vi "PH_IEEE1394Camera.PC Write Attribute.vi"(0 "i ref out":refnum<vi>, 1 "Attribute Name":string="N/A", 2 "Wanted Num":dbl, 3 "Wanted String":string="N/A", 4 "Wanted Bool":bool, 5 "error out":errorcluster) -> (14 "i ref out":refnum<vi>, 19 "error out":errorcluster)   [LabVIEW 2014, in "PH_IEEE1394Camera.lvlib"]
doc: "By this VI the cam attribute of Ibnterest is written to the hardware if the cam is off."
uses:
  PH_IEEE1394Camera.lvlib
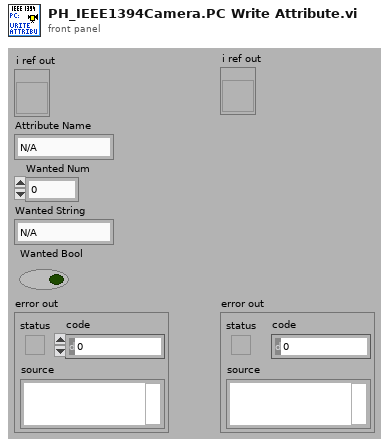
[diagram p1: front panel]
types:
  T1 = typedef "PH_IEEE1394Camera.lvlib/PH_IEEE1394Camera.i attribute.ctl" = cluster{"Gui Refs":cluster{"Brightness":refnum<vi>, "Shutter":refnum<vi>, "Gain":refnum<vi>, "Center of Gravity":refnum<vi>, "Supported Video Modes":refnum<vi>, "Trigger Polarity":refnum<vi>, "Trigger Mode":refnum<vi>, "Trigger Timeout":refnum<vi>, "Bit Depth":refnum<vi>, "Video Mode":refnum<vi>, "Top":refnum<vi>, "Bottom":refnum<vi>, "Left":refnum<vi>, "Right":refnum<vi>, "Set ROI to Maximum":refnum<vi>, "Camera Details":refnum<vi>, "Current Cam Attributes":refnum<vi>, "Attribute to set":refnum<vi>, "Num Value":refnum<vi>, "String Value":refnum<vi>, "Bool Value":refnum<vi>, "Set Cam Attribute":refnum<vi>}, "Cam":cluster{"IMAQ1394 Session":T2, "Camera Details":T3}, "Current Attributes":T4[], "Supported Video Modes ":cluster{"Video Mode":u32, "Video Mode Name":string}[], "Wanted Attributes":cluster{"Name":string, "Num Value":dbl, "String Value":string, "Boolean Value":bool}[], "Cam Attributes":T6}
  T2 = typedef "IMAQdx.ctl" = refnum<k21>
  T3 = typedef "PH_IEEE1394Camera.lvlib/PH_IEEE1394Camera.Cam Details.ctl" = cluster{"Model":string, "Serial Number":dbl, "Cam name (Machinery)":string, "Bus Type":string}
  T4 = typedef "PH_IEEE1394Camera.lvlib/PH_IEEE1394Camera.Cam Attribute.ctl" = cluster{"Information":cluster{"Type":T5, "Readable":bool, "Writable":bool, "Name":string}, "Num Value":dbl, "String Value":string, "Maximum":dbl, "Minimum":dbl, "Units":string, "Description":string, "EnumStrings[]":string[], "EnumValues[]":u32[], "Boolean Value":bool}
  T5 = typedef "NI_Vision_Acquisition_Software.lvlib/IMAQdx Attribute Type.ctl" = enum32{"U32", "I64", "DBL", "String", "Enum", "Bool", "Command"}
  T6 = typedef "PH_IEEE1394Camera.lvlib/PH_IEEE1394Camera.Relevant Cam Attributes.ctl" = cluster{"Video Mode":cluster{"Name":string, "Index":i32}, "Brightness":cluster{"Name":string, "Index":i32}, "Gain":cluster{"Name":string, "Index":i32}, "Shutter":cluster{"Name":string, "Index":i32}, "Trigger Pol":cluster{"Name":string, "Index":i32}, "Trigger Mode":cluster{"Name":string, "Index":i32}, "Timeout":cluster{"Name":string, "Index":i32}, "Bit Depth":cluster{"Name":string, "Index":i32}, "Pixel Bits":cluster{"Name":string, "Index":i32}, "Pixel Bytes":cluster{"Name":string, "Index":i32}, "Left":cluster{"Name":string, "Index":i32}, "Right":cluster{"Name":string, "Index":i32}, "Top":cluster{"Name":string, "Index":i32}, "Bottom":cluster{"Name":string, "Index":i32}}
  T7 = cluster{"Name":string, "Num Value":dbl, "String Value":string, "Boolean Value":bool}
  T8 = cluster{"Name":string, "Num Value":dbl, "String Value":string, "Boolean Value":bool}[]
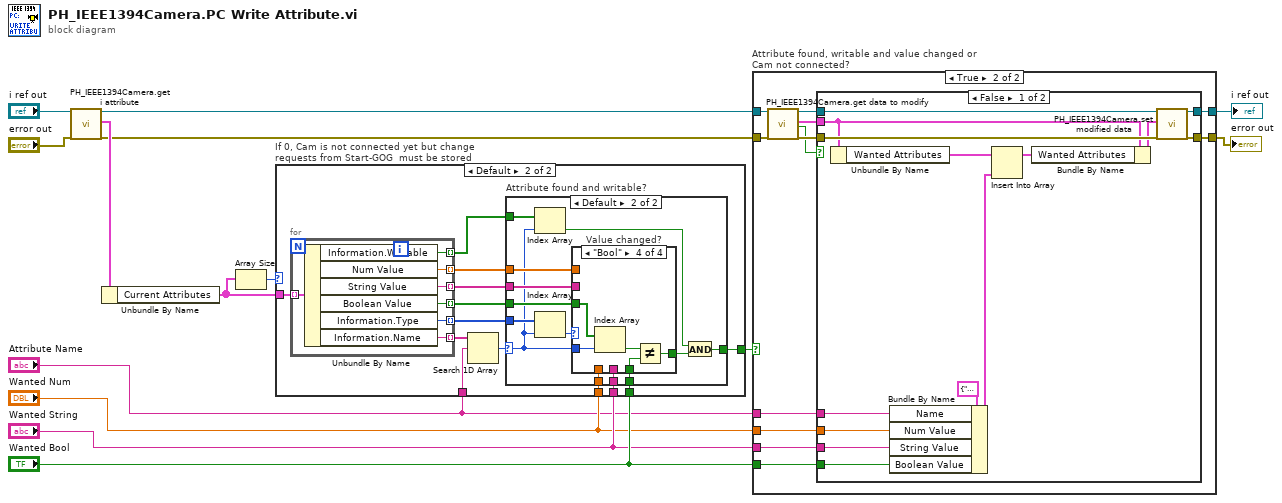
[diagram p0: block diagram]
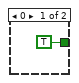
[diagram p2: hidden frame]
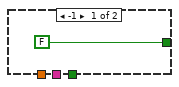
[diagram p3: hidden frame]
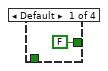
[diagram p4: hidden frame]
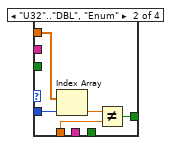
[diagram p5: hidden frame]
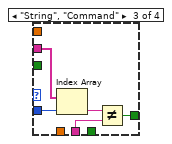
[diagram p6: hidden frame]
diagram:
  n1 = call "PH_IEEE1394Camera.get i attribute.vi"("i ref in"="i ref out", "error in (no error)"="error out") -> ("i ref out"=w11:refnum<vi>, "i attribute"=w12:T1, "error out"=w10:errorcluster)  [unwired: 15 in]
  n2 = Unbundle By Name(w12) -> ("Current Attributes"=w7:T4[])
  n3 = Array Size(array=w7) -> (size(s)=w4:i32)
  n4 = case "If 0, Cam is not connected yet but change requests from Start-GOG  must be stored" shown="Default" w4 {
    tunnel: w7 -> [_ w23]
    tunnel: [TRUE w22] -> w6
    tunnel: "Wanted Bool" -> [_ w20]
    tunnel: "Wanted String" -> [_ w19]
    tunnel: "Wanted Num" -> [_ w18]
    tunnel: "Attribute Name" -> [_ w17]
    frame 0 {
    }
    frame Default {
      n5 = for {
        tunnel: w23 -> [w65] mode=indexing
        tunnel: [w64] -> w21 mode=indexing
        tunnel: [w63] -> w28 mode=indexing
        tunnel: [w62] -> w27 mode=indexing
        tunnel: [w61] -> w26 mode=indexing
        tunnel: [w60] -> w25 mode=indexing
        tunnel: [w59] -> w24 mode=indexing
        n6 = Unbundle By Name(w65) -> ("Information.Writable"=w59:bool, "Num Value"=w62:dbl, "String Value"=w61:string, "Boolean Value"=w60:bool, "Information.Type"=w63:T5, "Information.Name"=w64:string)
      }
      n7 = Search 1D Array(1D array=w21, element=w17) -> (index of element=w16:i32)  [unwired: 1 in]
      n8 = case "Attribute found and writable?" shown="Default" w16 {
        selector: w16 -> [_ w30]
        tunnel: w28 -> [_ w42]
        tunnel: w27 -> [_ w41]
        tunnel: w26 -> [_ w40]
        tunnel: w25 -> [_ w39]
        tunnel: w24 -> [_ w38]
        tunnel: [FALSE w34] -> w22
        tunnel: w20 -> [_ w33]
        tunnel: w19 -> [_ w32]
        tunnel: w18 -> [_ w31]
        frame -1 {
        }
        frame Default {
          n9 = Index Array(array=w38, index=w30) -> (element=w35:bool)
          n10 = Index Array(array=w42, index=w30) -> (element=w37:T5)
          n11 = case "Value changed?" shown="\"Bool\"" w37 {
            tunnel: w41 -> [_ w48 _ _]
            tunnel: w30 -> [_ w47 w53 w58]
            tunnel: w31 -> [_ w45 _ _]
            tunnel: w32 -> [_ _ w49 _]
            tunnel: w33 -> [_ _ _ w54]
            tunnel: [FALSE w44 w51 w56] -> w36
            tunnel: w40 -> [_ _ w50 _]
            tunnel: w39 -> [_ _ _ w55]
            frame Default {
            }
            frame "U32".."DBL", "Enum" {
              n12 = Index Array(array=w48, index=w47) -> (element=w46:dbl)
              n13 = Not Equal?(x=w46, y=w45) -> (x != y?=w44:bool)
            }
            frame "String", "Command" {
              n14 = Index Array(array=w50, index=w53) -> (element=w52:string)
              n15 = Not Equal?(x=w52, y=w49) -> (x != y?=w51:bool)
            }
            frame "Bool" {
              n16 = Index Array(array=w55, index=w58) -> (element=w57:bool)
              n17 = Not Equal?(x=w57, y=w54) -> (x != y?=w56:bool)
            }
          }
          n18 = And(x=w35, y=w36) -> (x .and. y?=w34:bool)
        }
      }
    }
  }
  n19 = case "Attribute found, writable and value changed or Cam not connected?" shown="True" w6 {
    tunnel: w11 -> [w67 w79]
    tunnel: [w67 w77] -> w9
    tunnel: w10 -> [w66 w76]
    tunnel: [w66 w74] -> w8
    tunnel: "Wanted Bool" -> [_ w71]
    tunnel: "Wanted String" -> [_ w70]
    tunnel: "Wanted Num" -> [_ w69]
    tunnel: "Attribute Name" -> [_ w68]
    frame False {
    }
    frame True {
      n20 = call "PH_IEEE1394Camera.get data to modify.vi"("i ref in"=w79, "error in (no error)"=w76) -> ("i ref out"=w78:refnum<vi>, "i attribute"=w72:T1, "timed out"=w73:bool, "error out"=w75:errorcluster)  [unwired: 14 in]
      n21 = case shown="False" w73 {
        tunnel: w78 -> [w93 w94]
        tunnel: [w84 w94] -> w77
        tunnel: w75 -> [w92 w95]
        tunnel: [w83 w95] -> w74
        tunnel: w72 -> [w89 _]
        tunnel: w71 -> [w87 _]
        tunnel: w70 -> [w86 _]
        tunnel: w69 -> [w85 _]
        tunnel: w68 -> [w80 _]
        frame False {
          n22 = Unbundle By Name(w89) -> ("Wanted Attributes"=w90:T8)
          n23 = Bundle By Name(cluster=T7 {"Name"="", "Num Value"=0.0, "String Value"="", "Boolean Value"=FALSE} ("new element/subarray"), "Name"=w80, "Num Value"=w85, "String Value"=w86, "Boolean Value"=w87) -> (w81:T7)
          n24 = Insert Into Array(array=w90, new element=w81) -> (w88:T8)  [unwired: 1 in]
          n25 = Bundle By Name(cluster=w89, "Wanted Attributes"=w88) -> (w91:T1)
          n26 = call "PH_IEEE1394Camera.set modified data.vi"("i ref in"=w93, "i attribute"=w91, "error in (no error)"=w92) -> ("i ref out"=w84:refnum<vi>, "error out"=w83:errorcluster)  [unwired: 15 in]
        }
        frame True {
        }
      }
    }
  }
  "i ref out" <- w9
  "error out" <- w8
